vi "pump calibration.vi"(4 "pump cal command":T2=enum."Save default values", 5 "STAMP intercept":dbl, 6 "STAMP slope":dbl=2.52, 7 "flow rate":dbl[unit], 8 "Pump Calibration in":T1) -> (0 "STAMP intercept out":dbl, 1 "STAMP slope out":dbl=2.52, 2 "modified flow rate":dbl[unit], 3 "Pump Calibration out":T1)   [LabVIEW 2012]
uses:
  <vilib>/Utility/config.llb/NI_LVConfig.lvlib
  <vilib>/Utility/config.llb/Read Key (Double).vi
  <vilib>/Utility/config.llb/Write Key (Double).vi
  calibration commands.ctl
  calibration values.ctl
panel:
  in  "Pump Calibration default":T1={"target 1"=0.0, "target 2"=1e-06, "measured 1"=0.0, "measured 2"=1e-06}
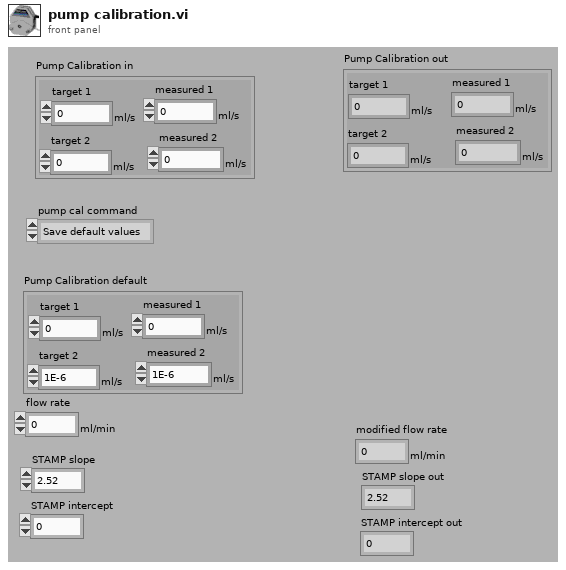
[diagram p1: front panel]
types:
  T1 = typedef "calibration values.ctl" = cluster{"target 1":dbl[unit], "target 2":dbl[unit], "measured 1":dbl[unit], "measured 2":dbl[unit]}
  T2 = typedef "calibration commands.ctl" = enum16{"Get ini Path", "Save default values", "Save new calibration", "Read calibration", "Apply calibration", "Read STAMP mb", "Write STAMP mb"}
  T3 = typedef "NI_LVConfig.lvlib/Config Data RefNum.ctl" = refnum<k1>
  T4 = cluster{"[0]":dbl[unit], "[1]":dbl[unit], "[2]":dbl[unit], "[3]":dbl[unit]}
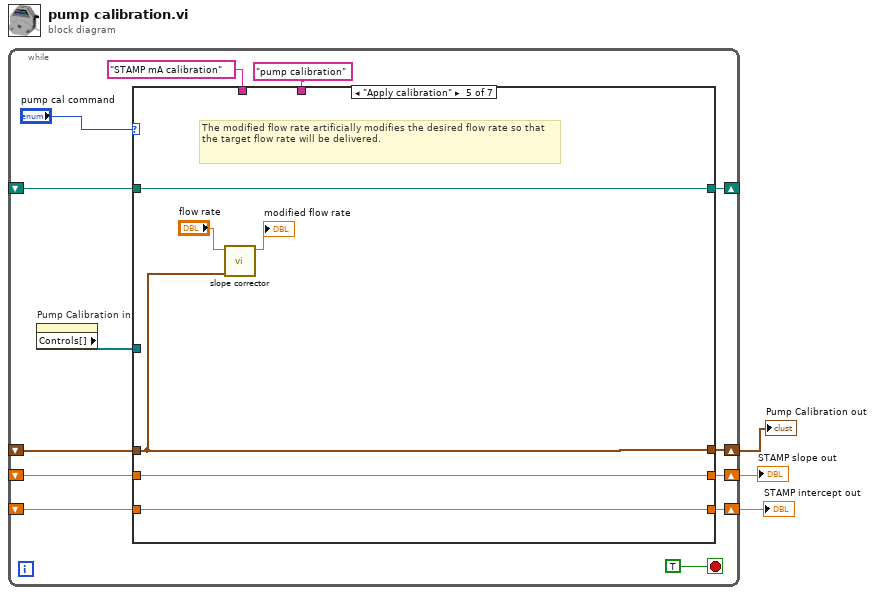
[diagram p0: block diagram]
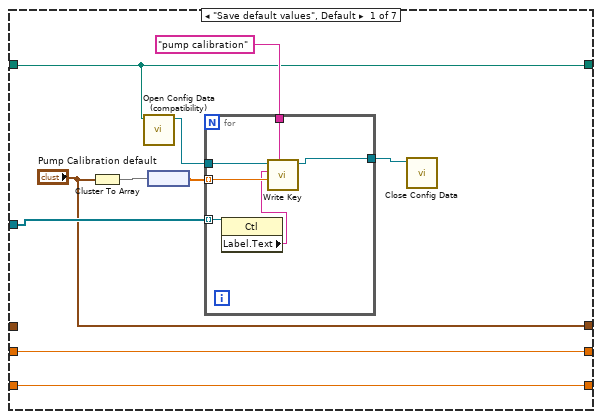
[diagram p2: hidden frame]
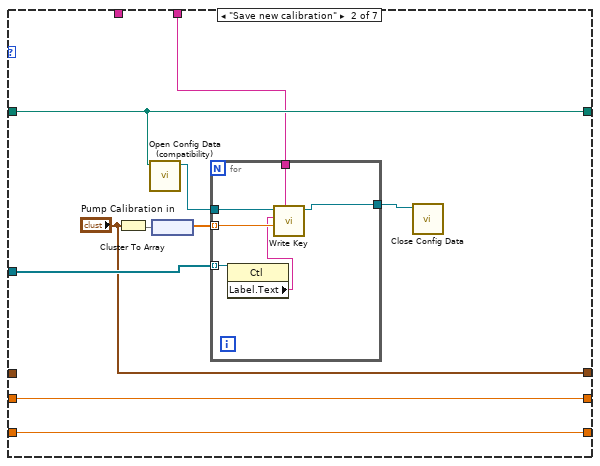
[diagram p3: hidden frame]
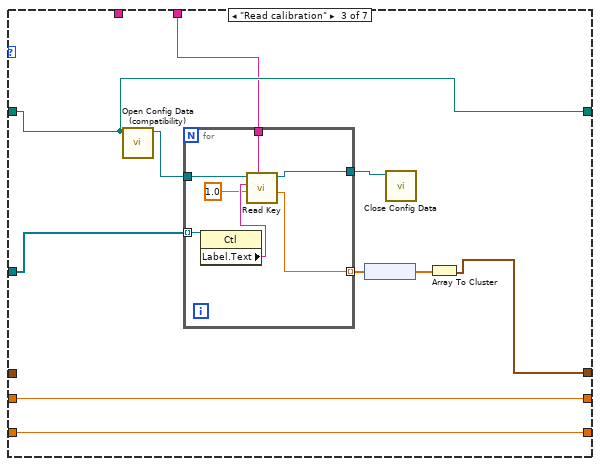
[diagram p4: hidden frame]
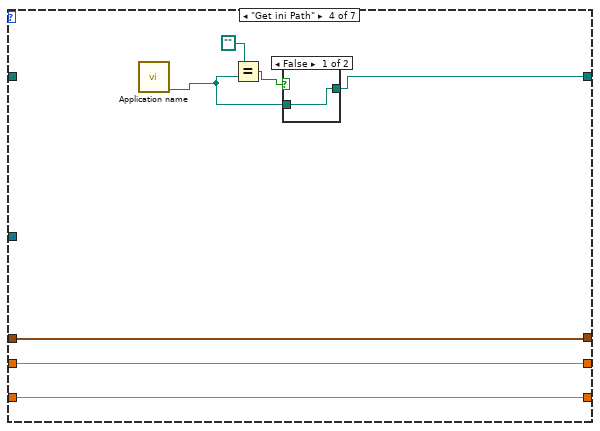
[diagram p5: hidden frame]
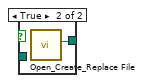
[diagram p6: hidden frame]
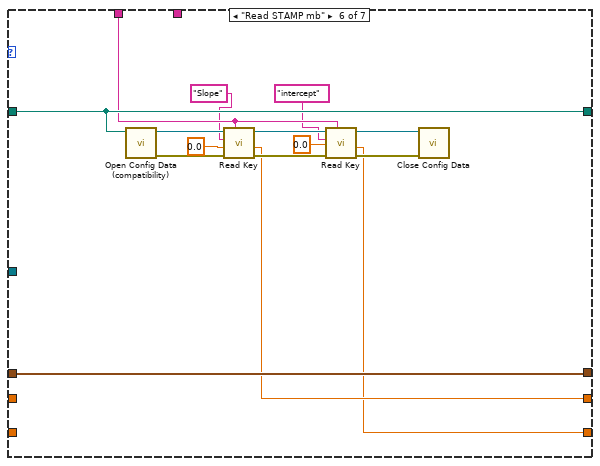
[diagram p7: hidden frame]
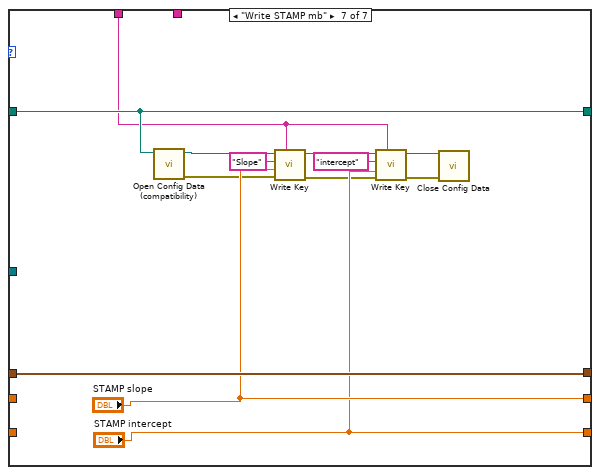
[diagram p8: hidden frame]
diagram:
  n1 = while {
    shift-right: [w13] -> _
    shift-left: _ -> [w15]
    shift-right: [w11] -> w1
    shift-left: _ -> [w10]
    shift-right: [w9] -> w2
    shift-left: _ -> [w7]
    shift-right: [w8] -> w3
    shift-left: _ -> [w6]
    stop <- TRUE stop-if-true
    n2 = property on="Pump Calibration in" class="Clust (strict)"() -> ("Controls[]"=w14:refnum<vi>[])  [unwired: 2 in, 2 out]
    n3 = case shown="\"Apply calibration\"" "pump cal command" {
      tunnel: w15 -> [w22 w40 w54 _ w79 w94 w107]
      tunnel: w14 -> [w21 w39 w55 _ _ _ _]
      tunnel: [w22 w40 w54 w70 w79 w94 w107] -> w13
      tunnel: ["Pump Calibration default" "Pump Calibration in" w53 w69 w80 w95 w108] -> w11
      tunnel: w10 -> [_ _ _ w69 w80 w95 w108]
      tunnel: [w18 w35 w51 w68 w76 w82 "STAMP slope"] -> w9
      tunnel: [w17 w34 w50 w67 w75 w81 "STAMP intercept"] -> w8
      tunnel: w7 -> [w18 w35 w51 w68 w76 _ _]
      tunnel: w6 -> [w17 w34 w50 w67 w75 _ _]
      tunnel: "STAMP mA calibration" ("section") -> [_ _ _ _ _ w85 w96]
      tunnel: "pump calibration" ("section") -> [_ w33 w49 _ _ _ _]
      frame "Save default values", Default {
        n4 = Cluster To Array(cluster="Pump Calibration default") -> (array=w25:dbl[unit][])
        n5 = call <vilib>:"Open Config Data (compatibility).vi"("configuration file path"=w22) -> ("refnum"=w26:T3)  [unwired: 8 in, 2 out]
        n6 = node(w25) -> (w19:dbl[])
        n7 = for {
          tunnel: w26 -> [w32]
          tunnel: w19 -> [w31] mode=indexing
          tunnel: w21 -> [w30] mode=indexing
          tunnel: "pump calibration" ("section") -> [w28]
          tunnel: [w27] -> w23
          n8 = property class="Ctl"(reference=w30) -> ("Label.Text"=w29:string)  [unwired: 1 in, 2 out]
          n9 = call-poly <vilib>:"Write Key.vi"("section"=w28, "value"=w31, "key"=w29, "refnum"=w32) -> ("refnum out"=w27:T3)  [unwired: 5 in, 2 out]
        }
        n10 = call <vilib>:"Close Config Data.vi"("refnum"=w23) -> ()  [unwired: 9 in, 2 out]
      }
      frame "Save new calibration" {
        n11 = Cluster To Array(cluster="Pump Calibration in") -> (array=w36:dbl[unit][])
        n12 = call <vilib>:"Open Config Data (compatibility).vi"("configuration file path"=w40) -> ("refnum"=w42:T3)  [unwired: 8 in, 2 out]
        n13 = node(w36) -> (w37:dbl[])
        n14 = for {
          tunnel: w42 -> [w48]
          tunnel: w37 -> [w47] mode=indexing
          tunnel: w39 -> [w46] mode=indexing
          tunnel: w33 -> [w44]
          tunnel: [w43] -> w41
          n15 = property class="Ctl"(reference=w46) -> ("Label.Text"=w45:string)  [unwired: 1 in, 2 out]
          n16 = call-poly <vilib>:"Write Key.vi"("section"=w44, "value"=w47, "key"=w45, "refnum"=w48) -> ("refnum out"=w43:T3)  [unwired: 5 in, 2 out]
        }
        n17 = call <vilib>:"Close Config Data.vi"("refnum"=w41) -> ()  [unwired: 9 in, 2 out]
      }
      frame "Read calibration" {
        n18 = call <vilib>:"Open Config Data (compatibility).vi"("configuration file path"=w54) -> ("refnum"=w58:T3)  [unwired: 8 in, 2 out]
        n19 = for {
          tunnel: w58 -> [w65]
          tunnel: w55 -> [w64] mode=indexing
          tunnel: w49 -> [w62]
          tunnel: [w61] -> w57
          tunnel: [w59] -> w56 mode=indexing
          n20 = property class="Ctl"(reference=w64) -> ("Label.Text"=w63:string)  [unwired: 1 in, 2 out]
          n21 = call-poly <vilib>:"Read Key.vi"("section"=w62, "default value"=1.0 ("target 1"), "key"=w63, "refnum"=w65) -> ("value"=w59:dbl, "refnum out"=w61:T3)  [unwired: 4 in, 2 out]
        }
        n22 = node(w56) -> (w52:dbl[unit][])
        n23 = call <vilib>:"Close Config Data.vi"("refnum"=w57) -> ()  [unwired: 9 in, 2 out]
        n24 = Array To Cluster(array=w52) -> (cluster=w53:T4)
      }
      frame "Get ini Path" {
        n25 = call "Application name.vi"() -> ("Ini file path"=w66:path)  [unwired: 4 in, 3 out]
        n26 = Equal?(x=path "", y=w66) -> (x = y?=w72:bool)
        n27 = case shown="False" w72 {
          tunnel: [w73 w74] -> w70
          tunnel: w66 -> [w73 _]
          frame False {
          }
          frame True {
            n28 = call <vilib>:"Open_Create_Replace File.vi"() -> ("new file path"=w74:path)  [unwired: 8 in, 3 out]
          }
        }
      }
      frame "Apply calibration" {
        # "The modified flow rate artificially modifies the desired flow rate so that the target flow rate will be delivered."
        n29 = call "slope corrector.vi"("Pump Calibration"=w80, "flow rate"="flow rate") -> ("modified flow rate"=→"modified flow rate":dbl[unit])  [unwired: 9 in]
      }
      frame "Read STAMP mb" {
        n30 = call <vilib>:"Open Config Data (compatibility).vi"("configuration file path"=w94) -> ("error out"=w90:errorcluster, "refnum"=w93:T3)  [unwired: 8 in, 1 out]
        n31 = call-poly <vilib>:"Read Key.vi"("section"=w85, "error in (no error)"=w90, "default value"=0.0 ("STAMP slope"), "key"="Slope", "refnum"=w93) -> ("error out"=w89:errorcluster, "value"=w82:dbl, "refnum out"=w92:T3)  [unwired: 3 in, 1 out]
        n32 = call-poly <vilib>:"Read Key.vi"("section"=w85, "error in (no error)"=w89, "default value"=0.0 ("STAMP intercept"), "key"="intercept", "refnum"=w92) -> ("error out"=w88:errorcluster, "value"=w81:dbl, "refnum out"=w91:T3)  [unwired: 3 in, 1 out]
        n33 = call <vilib>:"Close Config Data.vi"("error in (no error)"=w88, "refnum"=w91) -> ()  [unwired: 8 in, 2 out]
      }
      frame "Write STAMP mb" {
        n34 = call <vilib>:"Open Config Data (compatibility).vi"("configuration file path"=w107) -> ("error out"=w99:errorcluster, "refnum"=w106:T3)  [unwired: 8 in, 1 out]
        n35 = call-poly <vilib>:"Write Key.vi"("section"=w96, "error in (no error)"=w99, "value"="STAMP slope", "key"="Slope", "refnum"=w106) -> ("error out"=w98:errorcluster, "refnum out"=w104:T3)  [unwired: 4 in, 1 out]
        n36 = call-poly <vilib>:"Write Key.vi"("section"=w96, "error in (no error)"=w98, "value"="STAMP intercept", "key"="intercept", "refnum"=w104) -> ("error out"=w97:errorcluster, "refnum out"=w102:T3)  [unwired: 4 in, 1 out]
        n37 = call <vilib>:"Close Config Data.vi"("error in (no error)"=w97, "refnum"=w102) -> ()  [unwired: 8 in, 2 out]
      }
    }
  }
  "STAMP slope out" <- w2
  "STAMP intercept out" <- w3
  "Pump Calibration out" <- w1
